vi "tcp test.vi"() -> ()   [LabVIEW 2013]
panel:
  out "data out":string
  out "数据输出":string
  in  "布尔":bool=TRUE
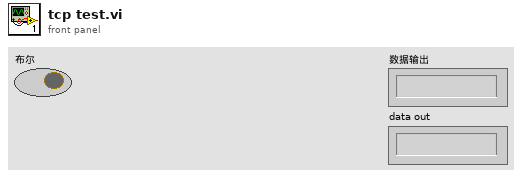
[diagram p1: front panel]
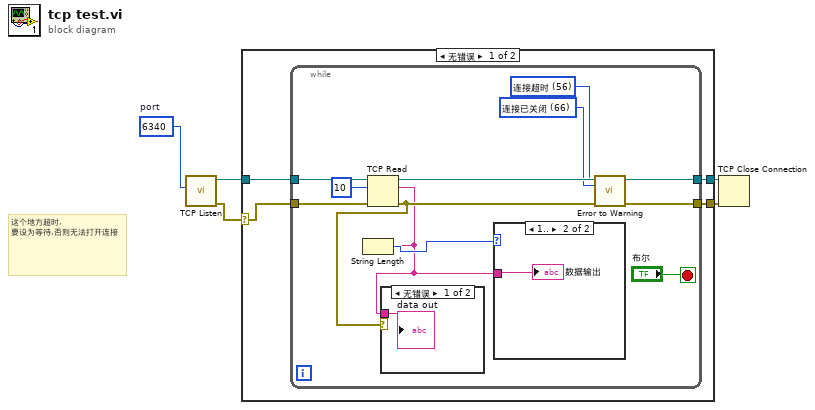
[diagram p0: block diagram]
diagram:
  w2 = u16 6340  # port
  # "这个地方超时, 要设为等待,否则无法打开连接"
  n1 = call <vilib>:"TCP Listen.vi"("port"=w2) -> ("error out"=w1:errorcluster, "connection ID"=w3:refnum<k5>)  [unwired: 6 in, 3 out]
  n2 = case shown="无错误" w1 {
    selector: w1 -> [w6 w23]
    tunnel: [w9 w24] -> w5
    tunnel: [w8 w23] -> w4
    tunnel: w3 -> [w7 w24]
    frame No Error {
      n3 = while {
        tunnel: w7 -> [w20]
        tunnel: w6 -> [w16]
        tunnel: [w17] -> w9
        tunnel: [w15] -> w8
        stop <- "布尔" stop-if-true
        w13 = 66 items=["无错误", "参数错误", "内存已满", "超出区域", "文件结束", "文件已打开", "一般文件IO错误", "未找到文件", "文件权限错误", "磁盘已满", "路径副本", "打开过多文件", "未启用", "未找到资源文件", "无法添加资源", "未找到资源", "未找到图像", "图像内存错误", "画笔不存在", "配置错误类型", "配置未找到解析段", "配置解析错误", "配置内存错误", "错误外部代码格式", "错误外部代码偏移量", "外部代码不存在", "空窗口", "销毁窗口错误", "空菜单", "打印已中止", "错误打印记录", "打印驱动程序错误", "打印时窗口错误", "打印时内存错误", "打印对话框错误", "一般打印错误", "无效设备引用句柄", "设备未找到", "设备参数错误", "设备单位错误", "无法打开设备", "设备调用已中止", "一般错误", "用户已取消", "对象ID过低", "对象ID过高", "对象不在堆中", "未知的堆", "错误DefProc ID", "DefProc不在表格中", "范围外信息", "空方法", "未知信息", "不支持管理器调用", "错误地址", "连接过程中", "连接超时", "连接过程中", "不支持网络属性", "网络错误", "正在使用的地址", "系统缺少内存", "连接已中止", "连接已拒绝", "连接未建立", "连接已建立", "连接已关闭", "初始化错误（交互应用程序管理器）", "错误事件发生", "等待无约束事件发生处理程序", "事件发生队列溢出", "错误路径", "未发出信号量", "未识别类型（交互应用程序管理器）"] ("2nd Error to Convert")
        w14 = 56 items=["无错误", "参数错误", "内存已满", "超出区域", "文件结束", "文件已打开", "一般文件IO错误", "未找到文件", "文件权限错误", "磁盘已满", "路径副本", "打开过多文件", "未启用", "未找到资源文件", "无法添加资源", "未找到资源", "未找到图像", "图像内存错误", "画笔不存在", "配置错误类型", "配置未找到解析段", "配置解析错误", "配置内存错误", "错误外部代码格式", "错误外部代码偏移量", "外部代码不存在", "空窗口", "销毁窗口错误", "空菜单", "打印已中止", "错误打印记录", "打印驱动程序错误", "打印时窗口错误", "打印时内存错误", "打印对话框错误", "一般打印错误", "无效设备引用句柄", "设备未找到", "设备参数错误", "设备单位错误", "无法打开设备", "设备调用已中止", "一般错误", "用户已取消", "对象ID过低", "对象ID过高", "对象不在堆中", "未知的堆", "错误DefProc ID", "DefProc不在表格中", "范围外信息", "空方法", "未知信息", "不支持管理器调用", "错误地址", "连接过程中", "连接超时", "连接过程中", "不支持网络属性", "网络错误", "正在使用的地址", "系统缺少内存", "连接已中止", "连接已拒绝", "连接未建立", "连接已建立", "连接已关闭", "初始化错误（交互应用程序管理器）", "错误事件发生", "等待无约束事件发生处理程序", "事件发生队列溢出", "错误路径", "未发出信号量", "未识别类型（交互应用程序管理器）"] ("1st Error to Convert")
        n4 = TCP Read(connection ID=w20, bytes to read=10 ("读取的字节"), error in (no error)=w16) -> (connection ID out=w17:refnum<k5>, data out=w10:string, error out=w11:errorcluster)  [unwired: 2 out]
        n5 = String Length(string=w10) -> (length=w12:i32)
        n6 = case shown="无错误" w11 {
          tunnel: w10 -> [w21 _]
          frame No Error {
            "data out" <- w21
          }
          frame Error {
          }
        }
        n7 = case shown="1.." w12 {
          tunnel: w10 -> [_ w22]
          frame 0, Default {
          }
          frame 1.. {
            "数据输出" <- w22
          }
        }
        n8 = call <vilib>:"Error to Warning.vi"("1st Error to Convert"=w14, "2nd Error to Convert"=w13, "error in"=w11) -> ("warning out"=w15:errorcluster)  [unwired: 12 in]
      }
    }
    frame Error {
    }
  }
  n9 = TCP Close Connection(connection ID=w5, error in (no error)=w4) -> ()  [unwired: 3 out]
